vi "stop vis.vi"(9 "Top Level VI's to stop":path[](array[path]), 11 "Panel VI's to stop":path[](array[path])) -> (0 "Stop VIs Error out":errorcluster[](array[cluster]))   [LabVIEW 2016, in "main.lvlib"]
doc: "stop vis.vi takes the sub-panel VI and Top Level VI paths (created by run vis.vi) and aborts them."
uses:
  main.lvlib
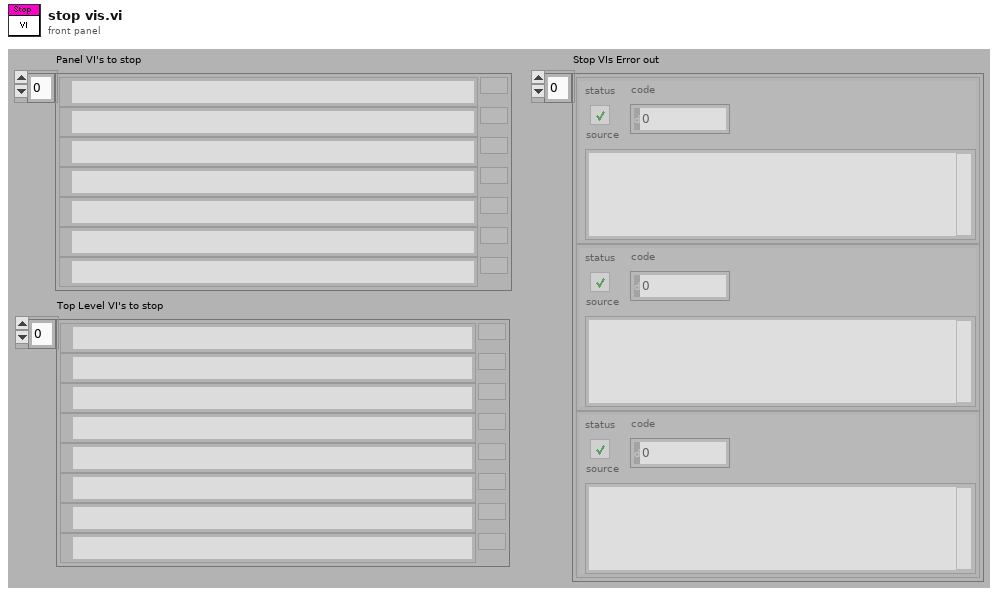
[diagram p1: front panel]
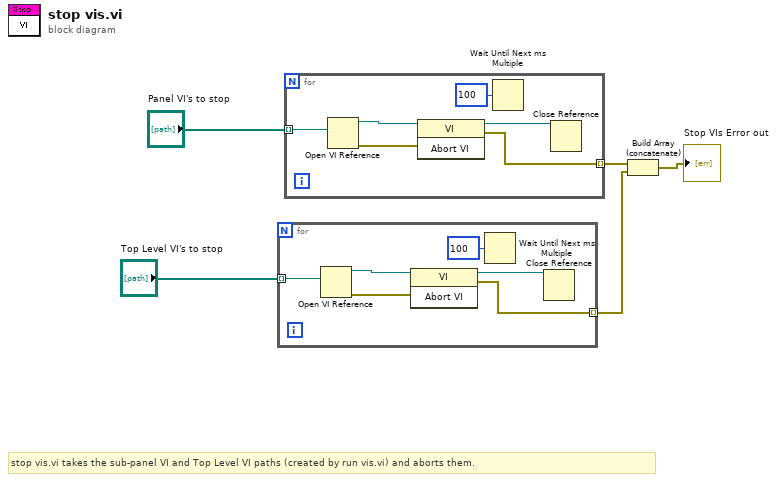
[diagram p0: block diagram]
diagram:
  # "stop vis.vi takes the sub-panel VI and Top Level VI paths (created by run vis.vi) and aborts them."
  n1 = for {
    tunnel: [w9] -> w1 mode=indexing
    tunnel: "Top Level VI's to stop" -> [w8] mode=indexing
    n2 = Open VI Reference(vi path=w8) -> (vi reference=w11:refnum<vi>, error out=w10:errorcluster)  [unwired: 2 in, 3 out]
    n3 = invoke class="VI" method="Abort VI"(reference=w11, error in=w10) -> (reference out=w7:refnum<vi>, error out=w9:errorcluster)  [unwired: 1 in, 1 out]
    n4 = Wait Until Next ms Multiple(millisecond multiple=u32 100) -> ()  [unwired: 1 out]
    n5 = Close Reference(reference=w7) -> ()  [unwired: 1 in, 1 out]
  }
  n6 = for {
    tunnel: [w15] -> w5 mode=indexing
    tunnel: "Panel VI's to stop" -> [w14] mode=indexing
    n7 = Open VI Reference(vi path=w14) -> (vi reference=w17:refnum<vi>, error out=w16:errorcluster)  [unwired: 2 in, 3 out]
    n8 = invoke class="VI" method="Abort VI"(reference=w17, error in=w16) -> (reference out=w13:refnum<vi>, error out=w15:errorcluster)  [unwired: 1 in, 1 out]
    n9 = Wait Until Next ms Multiple(millisecond multiple=u32 100) -> ()  [unwired: 1 out]
    n10 = Close Reference(reference=w13) -> ()  [unwired: 1 in, 1 out]
  }
  n11 = Build Array (concatenate)(w5, w1) -> (→"Stop VIs Error out":errorcluster[])
